vi "EnableAnalogPositionSettingValue.vi"(4 "error in (no error)":errorcluster, 7 "axis in":cluster{"keyHandle":u32, "nodeId":u16}={"keyHandle"=0, "nodeId"=1}) -> (0 "error out":errorcluster, 3 "axis out":cluster{"keyHandle":u32, "nodeId":u16}={"keyHandle"=0, "nodeId"=1})   [LabVIEW 2017, in "maxonEPOS.lvlib"]
doc: "<B>EnableAnalogPositionSetpoint</B> enables the analog position setpoint."
uses:
  Examples/maxonEPOS.lvlib
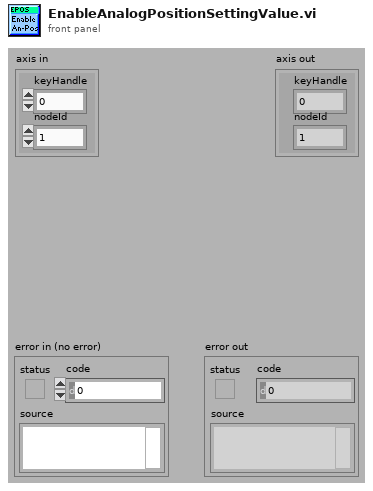
[diagram p1: front panel]
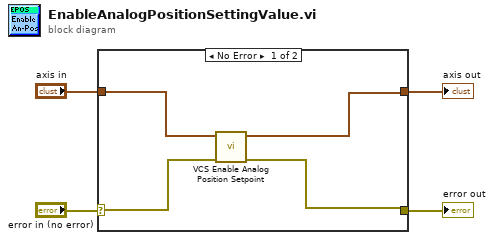
[diagram p0: block diagram]
diagram:
  n1 = case shown="No Error" "error in (no error)" {
    selector: "error in (no error)" -> [w6 w10]
    tunnel: [w7 w10] -> w3
    tunnel: [w8 w9] -> w2
    tunnel: "axis in" -> [w5 w9]
    frame No Error {
      n2 = call "VCS Enable Analog Position Setpoint.vi"("error in (no error)"=w6, "axis in"=w5) -> ("error out"=w7:errorcluster, "axis out"=w8:cluster{"keyHandle":u32, "nodeId":u16})  [unwired: 8 in]
    }
    frame Error {
    }
  }
  "error out" <- w3
  "axis out" <- w2
